vi "Get All Endpoints.vi"(8 "error in (no error)":errorcluster, 11 "Aliases Ref in":T1 format="%.0x") -> (0 "error out":errorcluster, 2 "Addressable Endpoints":string[](array[string]), 3 "Aliases Ref out":T1 format="%.0x")   [LabVIEW 2017, in "Routing and Faulting System Explorer.lvlib"]
uses:
  Routing and Faulting System Explorer.lvlib
  <vilib>/NI Veristand/Custom Device API/Custom Device Item Ref.ctl
  <vilib>/NI Veristand/Custom Device API/Custom Device API.lvlib
  Shared/Routing and Faulting Hardware API/Routing and Faulting Hardware API.lvlib
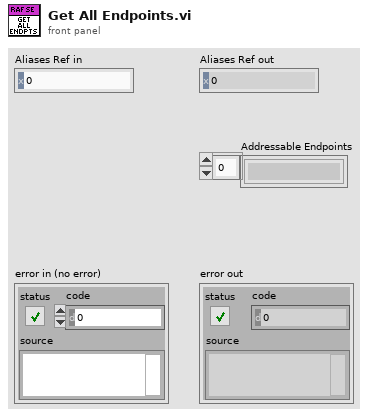
[diagram p1: front panel]
types:
  T1 = typedef "Custom Device API.lvlib/Custom Device Item Ref.ctl" = u64
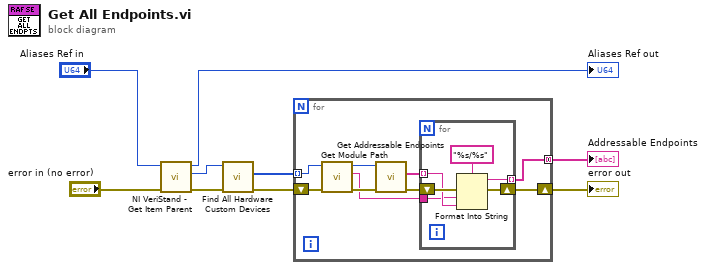
[diagram p0: block diagram]
diagram:
  n1 = call <vilib>:"NI VeriStand - Get Item Parent.vi"("error in (no error)"="error in (no error)", "Item Ref in"="Aliases Ref in") -> ("error out"=w7:errorcluster, "Parent Ref"=w6:T1, "Item Ref out"=→"Aliases Ref out":T1)  [unwired: 6 in, 1 out]
  n2 = call "Find All Hardware Custom Devices.vi"("error in (no error)"=w7, "Routing and Faulting Ref in"=w6) -> ("error out"=w4:errorcluster, "Hardware Refs"=w5:T1[])  [unwired: 7 in, 1 out]
  n3 = for {
    tunnel: w5 -> [w17] mode=indexing
    shift-right: [w13] -> w2
    shift-left: w4 -> [w18]
    tunnel: [w10] -> w3 mode=concatenating
    n4 = call "Get Module Path.vi"("error in (no error)"=w18, "Hardware Ref in"=w17) -> ("error out"=w15:errorcluster, "Resource"=w11:string, "Hardware Ref out"=w16:T1)  [unwired: 6 in, 1 out]
    n5 = call "Get Addressable Endpoints.vi"("error in (no error)"=w15, "Hardware Ref in"=w16) -> ("error out"=w14:errorcluster, "Addressable Endpoints"=w12:string[])  [unwired: 6 in, 2 out]
    n6 = for {
      shift-right: [w22] -> w13
      shift-left: w14 -> [w23]
      tunnel: w12 -> [w21] mode=indexing
      tunnel: w11 -> [w20]
      tunnel: [w19] -> w10 mode=indexing
      n7 = Format Into String(format string="%s/%s", error in=w23, w20, w21) -> (resulting string=w19:string, error out=w22:errorcluster)  [unwired: 1 in]
    }
  }
  "error out" <- w2
  "Addressable Endpoints" <- w3
